vi "getEvaluationStateList.vi"(8 "error in (no error)":errorcluster, 11 "VGS_RemoteControlClient in":refnum<class "VGS_RemoteControlClient.lvclass">) -> (0 "error out":errorcluster, 2 "getEvaluationStateList":refnum<k24>, 3 "VGS_RemoteControlClient out":refnum<class "VGS_RemoteControlClient.lvclass">)   [LabVIEW 2022 SP3, in "LV_VGS.lvlib" / "VGS_RemoteControlClient.lvclass"]
doc: "<B>Gets a list of EvaluatedObjectInfo objects for all evaluated scene elements. </B>\n\nThis method takes the remote handle and gets a list of EvaluatedObjectInfo objects for all evaluated elements currently in the scene. Alongside the evaluation state, this list will contain a path and a type for each object.\n\nAttention\nDepending on the size of the scene in VGStudio (MAX) and the number of evaluated objects, execution of this method can take some time! \nParameters\nhandle A valid remote handle. \n\nEmit error RemoteControlServiceIsNotAvailableException if the remote control service doesn't run. \nEmit error TooManyElementsInScene if the scene is too large to be handled. \nEmit error GenericRemoteControlErrorException if an internal error occurs.\nEmit error InvalidRemoteHandleException if the remote handle is not valid."
uses:
  VGS_RemoteControlClient.lvclass
  VGS_RemoteControlClient.lvclass/VGS_RemoteControlClient.ctl
  C:/Users/Andrey/Documents/GitHub/LV_VGS/vgs_project.dll
  vgs_project.dll
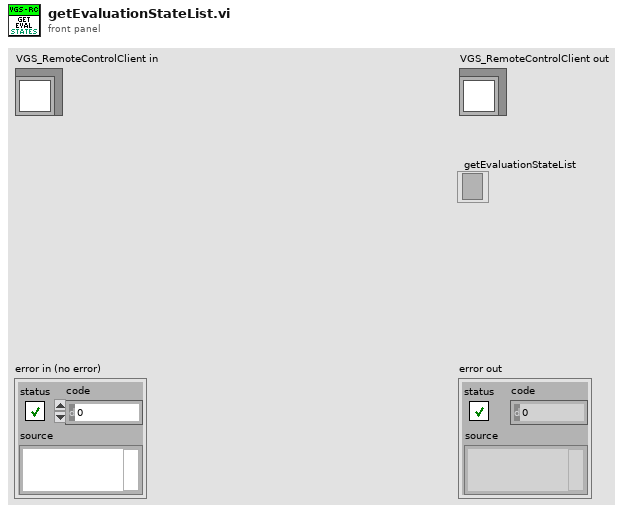
[diagram p1: front panel]
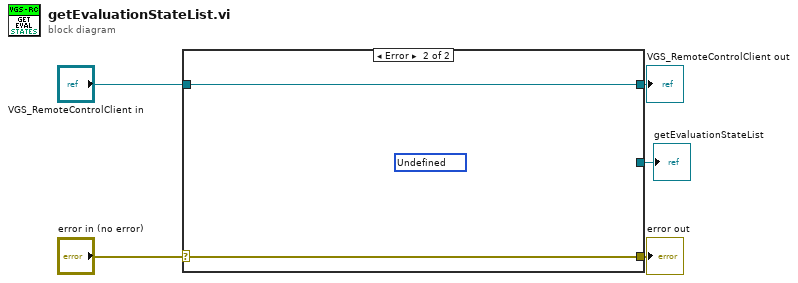
[diagram p0: block diagram]
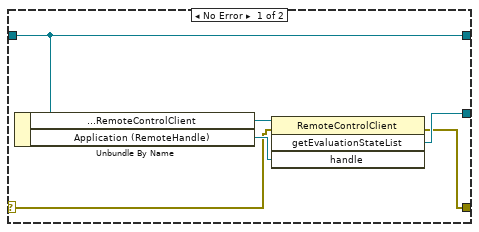
[diagram p2: hidden frame]
diagram:
  n1 = case shown="Error" "error in (no error)" {
    selector: "error in (no error)" -> [w7 w12]
    tunnel: [w6 w12] -> w4
    tunnel: [w11 w13] -> w2
    tunnel: "VGS_RemoteControlClient in" -> [w11 w13]
    tunnel: [w8 _] -> w1
    frame No Error {
      n2 = Unbundle By Name(w11) -> ("VGS.Project.Interop.RemoteControlClient"=w10:refnum<k24>, "Application (RemoteHandle)"=w9:refnum<k24>)
      n3 = invoke class="RemoteControlClient" method="getEvaluationStateList"(reference=w10, error in=w7, "handle"=w9) -> (error out=w6:errorcluster, "getEvaluationStateList"=w8:refnum<k24>)  [unwired: 1 in, 2 out]
    }
    frame Error {
      (unwired) 1448165568 items=["Undefined"=1448165568, "Valid"=1448165569, "OutOfTolerance"=1448165570, "InProgress"=1448165571, "NoTolerance"=1448165572] ("getEvaluationState")
    }
  }
  "error out" <- w4
  "VGS_RemoteControlClient out" <- w2
  "getEvaluationStateList" <- w1
